vi "Drive_Train_Control.vi"(11 "Command":enum16{"Run", "Init", "Auto"}(ring)) -> (3 "Value":T1=enum."Forward")   [LabVIEW 2016]
uses:
  <vilib>/Rock Robotics/WPI/Solenoid/WPI_SolenoidValue.ctl
  <vilib>/Rock Robotics/WPI/ThirdParty/CanMotor/TalonSRX/WPI_CANTalonSRX_APIControlMode.ctl
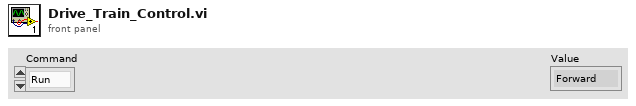
[diagram p1: front panel]
types:
  T1 = typedef "WPI_SolenoidValue.ctl" = enum16{"Off", "On", "Forward", "Reverse"}
  T2 = typedef "WPI_CANTalonSRX_APIControlMode.ctl" = enum8{"Percent VBus", "Speed", "Position", "Slave", "Unchanged / Invalid", "Voltage Compensation", "Current", "Motion Profile", "Motion Magic"}
  T3 = typedef "WPI_MotorControlDeviceRef.ctl" = cluster{"DeviceStatus":errorcluster, "Type":T4, "PWM":cluster{"PWM Channel":T5, "DeadBand":T6}, "CAN":cluster{"Device Number":u8, "SetOutput VI Ref":variant, "GetOutput VI Ref":variant, "Enable VI Ref":variant, "Disable VI Ref":variant, "Data":variant}, "Invert":bool}
  T4 = typedef "WPI_MotorControlType.ctl" = enum16{"PWM", "CAN"}
  T5 = typedef "FPGA_DIOPWMChannel.ctl" = enum8{"PWM 0", "PWM 1", "PWM 2", "PWM 3", "PWM 4", "PWM 5", "PWM 6", "PWM 7", "PWM 8", "PWM 9", "PWM MXP 0", "PWM MXP 1", "PWM MXP 2", "PWM MXP 3", "PWM MXP 4", "PWM MXP 5", "PWM MXP 6", "PWM MXP 7", "PWM MXP 8", "PWM MXP 9", "Invalid"}
  T6 = typedef "WPI_PWMDeadband.ctl" = cluster{"Name":string, "maxPositivePwm":i32, "minPositivePwm":i32, "centerPwm":i32, "maxNegativePwm":i32, "minNegativePwm":i32, "angularRange":u16}
  T7 = typedef "WPI_CANTalonSRX_GlobalStatus.ctl" = cluster{"Applied Throttle":dbl, "Module Enabled":bool, "CAN Error":errorcluster, "Closed Loop Error":dbl, "Forward Limit Switch Closed":bool, "Reverse Limit Switch Closed":bool, "Sensor Position":dbl, "Sensor Velocity":dbl, "Current":dbl, "Sticky Fault - Over Temp":bool, "Sticky Fault - Under Voltage":bool, "Sticky Fault - Forward Limit":bool, "Sticky Fault - Reverse Limit":bool, "Sticky Fault - Forward Soft Limit":bool, "Sticky Fault - Reverse Soft Limit":bool, "Brake is Enabled":bool, "Encoder Position":dbl, "Encoder Velocity":dbl, "Encoder Index Count":dbl, "Encoder A Pin State":bool, "Encoder B Pin State":bool, "Encoder Index Pin State":bool, "Analog In":dbl, "Analog In Velocity":dbl, "Temperature (C)":dbl, "Battery Voltage":dbl, "Control 5 Is Supported":bool, "Current Profile Slot Select":dbl, "Pos Div 8":bool, "Vel Div 4":bool, "Pulse Width Position":i32, "Pulse Width Velocity":i32, "Pulse Width Rise To Rise (us)":i32, "Pulse Width Rise To Fall (us)":i32, "Mot Prof Active Is Under Run":bool, "Mot Prof Active Has Under Run":bool, "Mot Prof Active Is Last":bool, "Mot Prof Active Velocity Only":bool, "Mot Prof Active Is Valid":bool, "Mot Prof Buffer Is Full":bool, "Mot Prof Active Profile Slot Select":i32, "Mot Prof NextID":i32, "Mot Prof Count":i32, "Mot Prof Active Velocity":dbl, "Mot Prof Active Position":dbl, "Mot Prof Output Enable":i32}
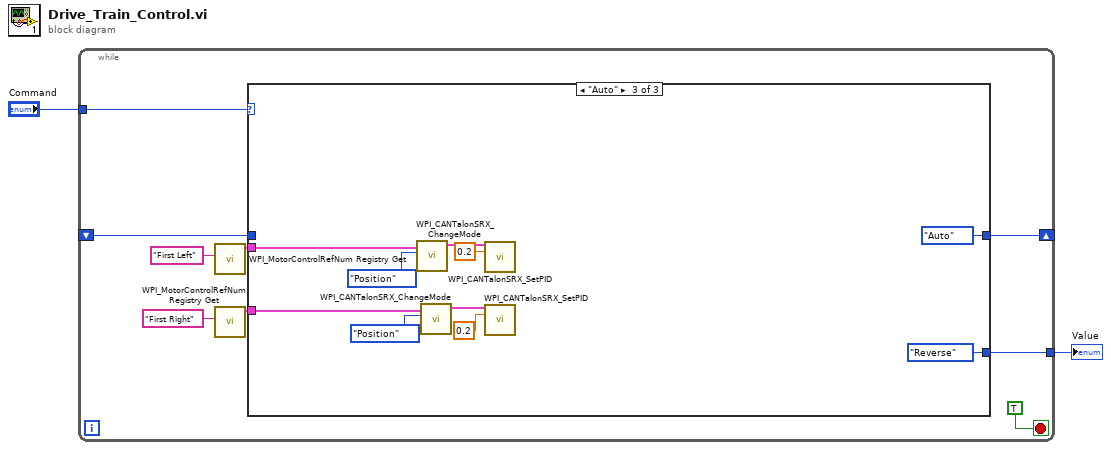
[diagram p0: block diagram]
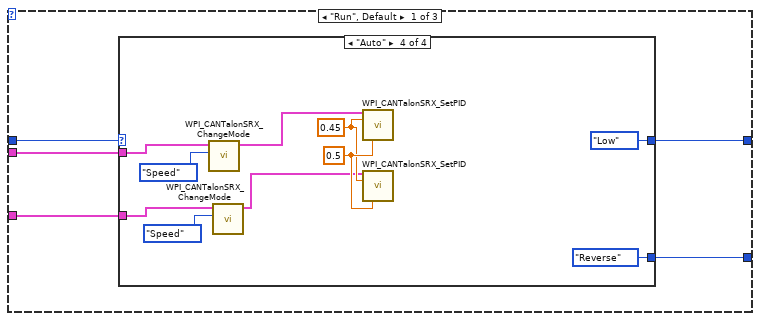
[diagram p2: hidden frame]
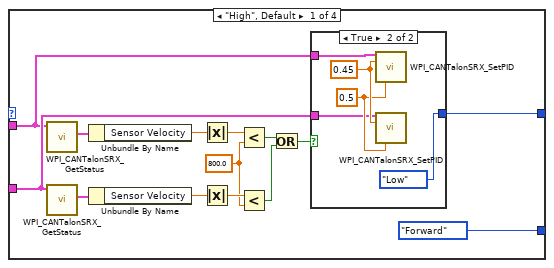
[diagram p3: hidden frame]
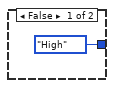
[diagram p4: hidden frame]
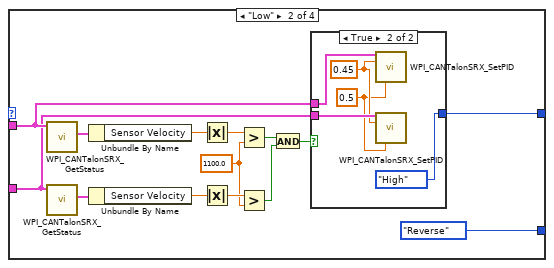
[diagram p5: hidden frame]
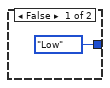
[diagram p6: hidden frame]
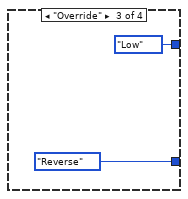
[diagram p7: hidden frame]
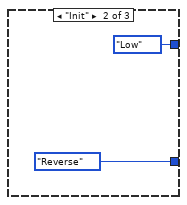
[diagram p8: hidden frame]
diagram:
  n1 = while {
    tunnel: "Command" -> [w10]
    tunnel: [w5] -> w1
    shift-right: [w4] -> _
    shift-left: _ -> [w3]
    stop <- TRUE stop-if-true
    n2 = call <vilib>:"WPI_MotorControlRefNum Registry Get.vi"("refnum name"="First Left") -> ("MotorControlDevRef"=w7:T3)  [unwired: 9 in, 1 out]
    n3 = call <vilib>:"WPI_MotorControlRefNum Registry Get.vi"("refnum name"="First Right") -> ("MotorControlDevRef"=w6:T3)  [unwired: 9 in, 1 out]
    n4 = case shown="\"Auto\"" w10 {
      tunnel: [w16 enum16{"High", "Low", "Override", "Auto"}."Low" enum16{"High", "Low", "Override", "Auto"}."Auto"] -> w4
      tunnel: w7 -> [w15 _ w80]
      tunnel: w6 -> [w14 _ w79]
      tunnel: [w13 WPI_SolenoidValue."Reverse" ("Value") WPI_SolenoidValue."Reverse" ("Value")] -> w5
      tunnel: w3 -> [w12 _ _]
      frame "Run", Default {
        n5 = case shown="\"Auto\"" w12 {
          tunnel: [w17 w40 enum16{"High", "Low", "Override", "Auto"}."Low" enum16{"High", "Low", "Override", "Auto"}."Low"] -> w16
          tunnel: w15 -> [w18 w39 _ w66]
          tunnel: w14 -> [w19 w38 _ w65]
          tunnel: [WPI_SolenoidValue."Forward" ("Value") WPI_SolenoidValue."Reverse" ("Value") WPI_SolenoidValue."Reverse" ("Value") WPI_SolenoidValue."Reverse" ("Value")] -> w13
          frame "High", Default {
            w24 = 800.0 ("y")
            n6 = call <vilib>:"WPI_CANTalonSRX_GetStatus.vi"("CAN Talon SRX Ref"=w18) -> ("Talon SRX Status"=w29:T7)  [unwired: 8 in, 2 out]
            n7 = call <vilib>:"WPI_CANTalonSRX_GetStatus.vi"("CAN Talon SRX Ref"=w19) -> ("Talon SRX Status"=w30:T7)  [unwired: 8 in, 2 out]
            n8 = Unbundle By Name(w29) -> ("Sensor Velocity"=w27:dbl)
            n9 = Unbundle By Name(w30) -> ("Sensor Velocity"=w28:dbl)
            n10 = Absolute Value(x=w27) -> (abs(x)=w26:dbl)
            n11 = Absolute Value(x=w28) -> (abs(x)=w25:dbl)
            n12 = Less?(x=w26, y=w24) -> (x < y?=w23:bool)
            n13 = Less?(x=w25, y=w24) -> (x < y?=w22:bool)
            n14 = Or(x=w23, y=w22) -> (x .or. y?=w21:bool)
            n15 = case shown="True" w21 {
              tunnel: [enum16{"High", "Low", "Override", "Auto"}."High" enum16{"High", "Low", "Override", "Auto"}."Low"] -> w17
              tunnel: w19 -> [_ w33]
              tunnel: w18 -> [_ w32]
              frame False {
              }
              frame True {
                w34 = 0.5 ("F")
                w35 = 0.45 ("P")
                n16 = call <vilib>:"WPI_CANTalonSRX_SetPID.vi"("CAN Talon SRX Ref"=w32, "P"=w35, "F"=w34) -> ()  [unwired: 11 in, 2 out]
                n17 = call <vilib>:"WPI_CANTalonSRX_SetPID.vi"("CAN Talon SRX Ref"=w33, "P"=w35, "F"=w34) -> ()  [unwired: 11 in, 2 out]
              }
            }
          }
          frame "Low" {
            w44 = 1100.0 ("y")
            n18 = call <vilib>:"WPI_CANTalonSRX_GetStatus.vi"("CAN Talon SRX Ref"=w39) -> ("Talon SRX Status"=w49:T7)  [unwired: 8 in, 2 out]
            n19 = call <vilib>:"WPI_CANTalonSRX_GetStatus.vi"("CAN Talon SRX Ref"=w38) -> ("Talon SRX Status"=w50:T7)  [unwired: 8 in, 2 out]
            n20 = Unbundle By Name(w49) -> ("Sensor Velocity"=w47:dbl)
            n21 = Unbundle By Name(w50) -> ("Sensor Velocity"=w48:dbl)
            n22 = Absolute Value(x=w47) -> (abs(x)=w46:dbl)
            n23 = Absolute Value(x=w48) -> (abs(x)=w45:dbl)
            n24 = Greater?(x=w46, y=w44) -> (0:w43:bool)
            n25 = Greater?(x=w45, y=w44) -> (0:w42:bool)
            n26 = And(x=w43, y=w42) -> (x .and. y?=w41:bool)
            n27 = case shown="True" w41 {
              tunnel: [enum16{"High", "Low", "Override", "Auto"}."Low" enum16{"High", "Low", "Override", "Auto"}."High"] -> w40
              tunnel: w39 -> [_ w55]
              tunnel: w38 -> [_ w54]
              frame False {
              }
              frame True {
                w52 = 0.5 ("F")
                w53 = 0.45 ("P")
                n28 = call <vilib>:"WPI_CANTalonSRX_SetPID.vi"("CAN Talon SRX Ref"=w55, "P"=w53, "F"=w52) -> ()  [unwired: 11 in, 2 out]
                n29 = call <vilib>:"WPI_CANTalonSRX_SetPID.vi"("CAN Talon SRX Ref"=w54, "P"=w53, "F"=w52) -> ()  [unwired: 11 in, 2 out]
              }
            }
          }
          frame "Override" {
          }
          frame "Auto" {
            w62 = 0.5 ("F")
            w61 = 0.45 ("P")
            n30 = call <vilib>:"WPI_CANTalonSRX_ChangeMode.vi"("Control Mode"=WPI_CANTalonSRX_APIControlMode."Speed", "CAN Talon SRX Ref"=w66) -> ("CAN Talon SRX Ref"=w60:T3)  [unwired: 8 in, 1 out]
            n31 = call <vilib>:"WPI_CANTalonSRX_ChangeMode.vi"("Control Mode"=WPI_CANTalonSRX_APIControlMode."Speed", "CAN Talon SRX Ref"=w65) -> ("CAN Talon SRX Ref"=w59:T3)  [unwired: 8 in, 1 out]
            n32 = call <vilib>:"WPI_CANTalonSRX_SetPID.vi"("CAN Talon SRX Ref"=w60, "P"=w61, "F"=w62) -> ()  [unwired: 11 in, 2 out]
            n33 = call <vilib>:"WPI_CANTalonSRX_SetPID.vi"("CAN Talon SRX Ref"=w59, "P"=w61, "F"=w62) -> ()  [unwired: 11 in, 2 out]
          }
        }
      }
      frame "Init" {
      }
      frame "Auto" {
        n34 = call <vilib>:"WPI_CANTalonSRX_ChangeMode.vi"("Control Mode"=WPI_CANTalonSRX_APIControlMode."Position", "CAN Talon SRX Ref"=w80) -> ("CAN Talon SRX Ref"=w76:T3)  [unwired: 8 in, 1 out]
        n35 = call <vilib>:"WPI_CANTalonSRX_ChangeMode.vi"("Control Mode"=WPI_CANTalonSRX_APIControlMode."Position", "CAN Talon SRX Ref"=w79) -> ("CAN Talon SRX Ref"=w75:T3)  [unwired: 8 in, 1 out]
        n36 = call <vilib>:"WPI_CANTalonSRX_SetPID.vi"("CAN Talon SRX Ref"=w76, "P"=0.2) -> ()  [unwired: 12 in, 2 out]
        n37 = call <vilib>:"WPI_CANTalonSRX_SetPID.vi"("CAN Talon SRX Ref"=w75, "P"=0.2) -> ()  [unwired: 12 in, 2 out]
      }
    }
  }
  "Value" <- w1
